vi "Init and Rotate array bool.vi"(5 "Reset":bool, 7 "Stop read":bool, 9 "Array size":i32=30, 11 "In":bool) -> (3 "Array":bool[](array[boolean]))   [LabVIEW 2019, in "Userlib.lvlib"]
uses:
  Userlib.lvlib
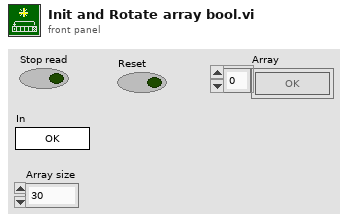
[diagram p1: front panel]
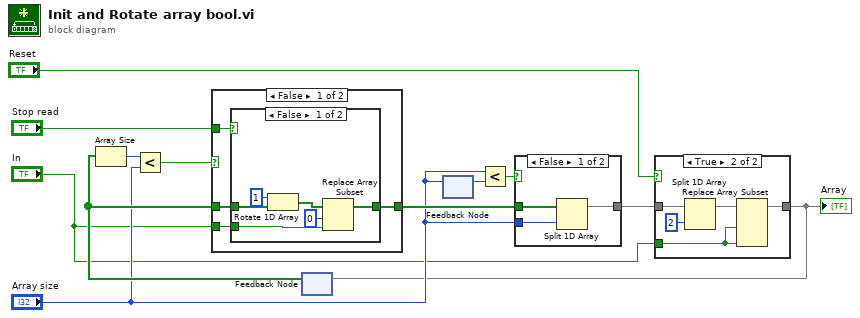
[diagram p0: block diagram]
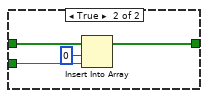
[diagram p3: hidden frame]
diagram:
  n1 = feedback #1() -> (w6:bool[])  [unwired: 1 in]
  n2 = Array Size(array=w6) -> (size(s)=w12:i32)
  n3 = Less?(x=w12, y="Array size") -> (x < y?=w2:bool)
  n4 = case shown="False" w2 {
    tunnel: [w14 w27] -> w7
    tunnel: "In" -> [w15 w24]
    tunnel: w6 -> [w16 w26]
    tunnel: "Stop read" -> [w13 _]
    frame False {
      n5 = case shown="False" w13 {
        tunnel: w16 -> [w19 w23]
        tunnel: w15 -> [w18 _]
        tunnel: [w17 w23] -> w14
        frame False {
          n6 = Rotate 1D Array(1:w19, 2:1 ("n")) -> (0:w21:bool[])
          n7 = Replace Array Subset(array=w21, new element=w18, index=0) -> (w17:bool[])
        }
        frame True {
        }
      }
    }
    frame True {
      n8 = Insert Into Array(array=w26, index=0, new element=w24) -> (w27:bool[])
    }
  }
  n9 = feedback #2() -> (w11:i32)  [unwired: 1 in]
  n10 = feedback-in #2("Array size") -> ()
  n11 = Less?(x="Array size", y=w11) -> (x < y?=w10:bool)
  n12 = case shown="False" w10 {
    tunnel: [w28 w31] -> w8
    tunnel: w7 -> [w30 w31]
    tunnel: "Array size" -> [w29 _]
    frame False {
      n13 = Split 1D Array(array=w30, index=w29) -> (first subarray=w28:bool[])  [unwired: 1 out]
    }
    frame True {
    }
  }
  n14 = case shown="True" "Reset" {
    tunnel: [w32 w34] -> w1
    tunnel: w8 -> [w32 w37]
    tunnel: "In" -> [_ w33]
    frame False {
    }
    frame True {
      n15 = Split 1D Array(array=w37, index=2) -> (first subarray=w36:bool[])  [unwired: 1 out]
      n16 = Replace Array Subset(array=w36, new element #1=w33, new element #2=w33) -> (w34:bool[])  [unwired: 2 in]
    }
  }
  "Array" <- w1
  n17 = feedback-in #1(w1) -> ()
